vi "Query Relay State.vi"(8 "error in":errorcluster, 11 "2525 in":refnum<class "2525.lvclass">) -> (0 "error out":errorcluster, 2 "Relay State":bool[](array[boolean]), 3 "2525 out":refnum<class "2525.lvclass">)   [LabVIEW 2019, in "2525.lvlib" / "2525.lvclass"]
uses:
  Library/2525.lvclass
  C:/Users/Public/Documents/Development/builds/Instruments/SwitchMatrix.lvlibp/SwitchMatrix.lvclass
  Library/2525.lvclass/2525.ctl
  <instrlib>/niSwitch/niSwitch.llb/niSwitch Relay Position.ctl
  Accessors/Read Local Resource.vi
  Accessors/Write Local Resource.vi
  builds/Instruments/SwitchMatrix.lvlibp/Accessors/Write Relay State.vi
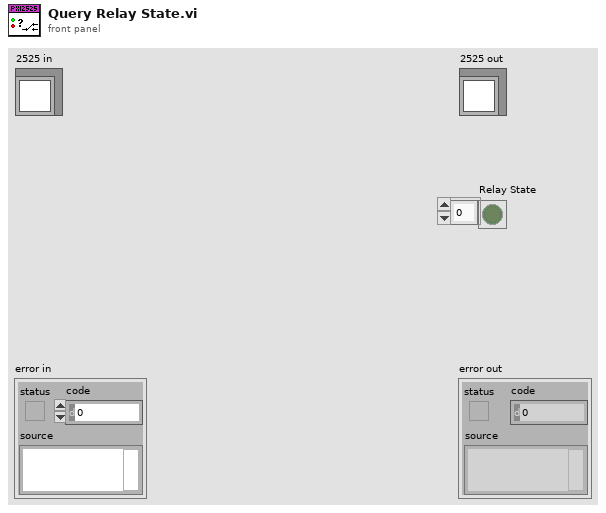
[diagram p1: front panel]
types:
  T1 = typedef "niSwitch Relay Position.ctl" = i32
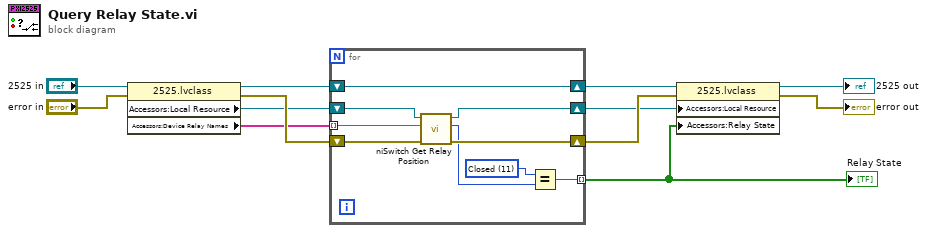
[diagram p0: block diagram]
diagram:
  n1 = property class="2525.lvclass"(reference="2525 in", error in="error in") -> (reference out=w10:refnum<class "2525.lvclass">, error out=w9:errorcluster, "Accessors:Local Resource"=w8:refnum<k15>, "Accessors:Device Relay Names"=w7:string[])
  n2 = for {
    shift-right: [w21] -> w3
    shift-left: w10 -> [w21]
    shift-right: [w16] -> w2
    shift-left: w9 -> [w18]
    shift-right: [w17] -> w1
    shift-left: w8 -> [w20]
    tunnel: w7 -> [w19] mode=indexing
    tunnel: [w13] -> w4 mode=indexing
    w14 = T1 11 items=["Open"=10, "Closed"=11] ("x")
    n3 = call <instrlib>:"niSwitch Get Relay Position.vi"("error in (no error)"=w18, "relay name"=w19, "instrument handle"=w20) -> ("error out"=w16:errorcluster, "position"=w15:T1, "instrument handle out"=w17:refnum<k15>)  [unwired: 6 in]
    n4 = Equal?(x=w14, y=w15) -> (x = y?=w13:bool)
  }
  "Relay State" <- w4
  n5 = property class="2525.lvclass"(reference=w3, error in=w2, "Accessors:Local Resource"=w1, "Accessors:Relay State"=w4) -> (reference out=→"2525 out":refnum<class "2525.lvclass">, error out=→"error out":errorcluster)
